vi "Sweep Control.vi"(0 "Scan control":T12=[{"Priority"=enum."Priority 1", "Scan name"=enum."OFF"}, {"Priority"=enum."Priority 0", "Scan name"=enum."DSA_freq"}, {"Priority"=enum."Priority 3", "Scan name"=enum."OFF"}, {"Priority"=enum."Priority 2", "Scan name"=enum."OFF"}], 1 "Scan parameters":T10=[{"DAQ Channel"=0, "Label"="\nappliedDC=", "Start"=-0.00372, "End"=0.00428, "Step"=5e-05, "Rate"=0.0, "VISA resource name"=""}, {"DAQ Channel"=3, "Label"="\nappliedField=", "Start"=0.3, "End"=0.0, "Step"=0.02, "Rate"=0.05, "VISA resource name"=""}, {"DAQ Channel"=3, "Label"="\nappliedVbg=", "Start"=-1.55, "End"=3.0, "Step"=0.015, "Rate"=2.0, "VISA resource name"=""}, {"DAQ Channel"=3, "Label"="\nappliedField=", "Start"=0.0, "End"=10000.0, "Step"=5000.0, "Rate"=0.0, "VISA resource name"=""}] {"Rate" format="%.2f"; "Step" format="%#_6p"; "End" format="%#_6p"; "Start" format="%#_6p"}, 3 "Comments":string="B sweep from 0.3T to 0T, 0.02T step\nDC sweep from -4mV to 4mV, 5uV step\nVbg = -5V\nVsg=40mV\nT<60mK\n\nI+/-: rightwire 1/2 200uV + DC sweep, f=9\nI2-: grounded on 4\nBase f=3\nV+/-: 5/7\nV2+/-: 4/28\nVsg: 6", 4 "Experiment folder name":string="21-SmallBsweep-DCsweep-rightdrive12-leftgrounded") -> ()   [LabVIEW 2016, in "Transport.lvclass"]
uses:
  Transport.lvclass
  Typedefs/ScanControl.ctl
  Typedefs/Cluster - ScanControl.ctl
  Typedefs/Enum - Priority.ctl
  Typedefs/Enum - Action.ctl
  Typedefs/ScanParamters.ctl
  Typedefs/Cluster - ScanParamters.ctl
  Typedefs/PostAction.ctl
  Typedefs/Enum - PostAction.ctl
  <userlib>/LevyLab/Lockin-Multichannel/Typedefs/AO-cluster.ctl
  <userlib>/LevyLab/Lockin-Multichannel/Typedefs/AO_Amp-array.ctl
  <userlib>/LevyLab/Lockin-Multichannel/Typedefs/AO_DC-array.ctl
  <userlib>/LevyLab/Lockin-Multichannel/Typedefs/AO_f-array.ctl
  <userlib>/LevyLab/Lockin-Multichannel/Typedefs/AO_phi-array.ctl
  <userlib>/LevyLab/Lockin-Multichannel/Typedefs/Function-array.ctl
  <userlib>/LevyLab/Lockin-Multichannel/Typedefs/Function-enum.ctl
  <userlib>/_OpenG.lib/array/array.llb/Empty 1D Array (Variant)__ogtk.vi
panel:
  in  "Channels: AO":T1={"AO amp (V)"=[0.0002, 0.0, 0.0, 0.0, 0.0, 0.0, 0.0, 0.0], "AO DC (V)"=[-0.004, 0.0, 0.04, 0.0, 0.0, 0.0, 0.0, 0.0], "AO f (Hz)"=[9.0, 3.0, 3.0, 3.0, 3.0, 3.0, 3.0, 3.0], "AO phi (deg)"=[0.0, 0.0, 0.0, 0.0, 0.0, 0.0, 0.0, 0.0], "function"=[enum."Sine Wave", enum."Sine Wave", enum."Sine Wave", enum."Sine Wave", enum."Sine Wave", enum."Sine Wave", enum."Sine Wave", enum."Sine Wave"]} {"AO f (Hz)" min=0.001 max=10000.0; "AO DC (V)" format="%#_6p"; "AO amp (V)" format="%#_6p"}
  in  "Experiment":enum16{"IV", "lockin_time", "Lockin_Vsg"}(ring)=enum."Lockin_Vsg"
  in  "Post action (indexing priority)":T8=[enum."Do Nothing", enum."Wait", enum."Do Nothing", enum."Do Nothing"]
  in  "Number of IV curves":i32=1
  # "if you use the lockin\nprogram remember to\nset BG/SG parameters in\n'lockin_Vsg_multichannel.vi'"
  # "Instructions: \n1, you can put multiple scan names in one priority.\n2 OFF has to put in last priority"
  # "0"
  # "1"
  # "2"
  # "3"
  # "4"
  # "5"
  # "6"
  # "7"
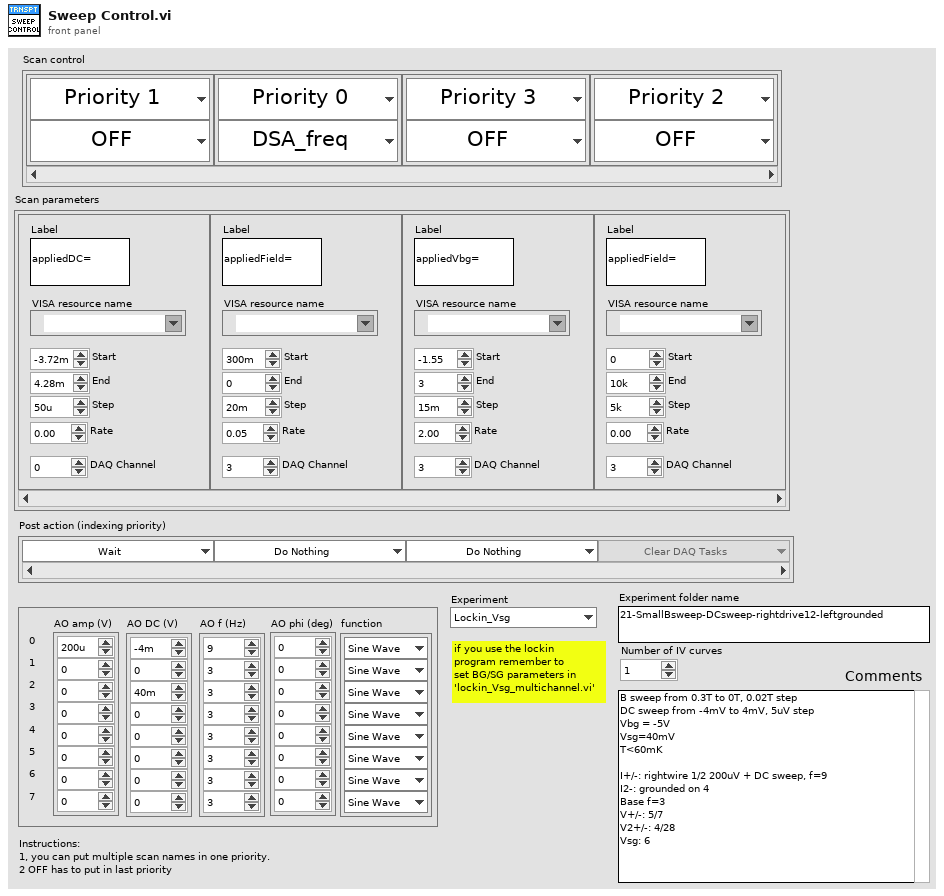
[diagram p1: front panel]
types:
  T1 = typedef "AO-cluster.ctl" = cluster{"AO amp (V)":T2, "AO DC (V)":T3, "AO f (Hz)":T4, "AO phi (deg)":T5, "function":T6}
  T2 = typedef "AO_Amp-array.ctl" = dbl[]
  T3 = typedef "AO_DC-array.ctl" = dbl[]
  T4 = typedef "AO_f-array.ctl" = dbl[]
  T5 = typedef "AO_phi-array.ctl" = dbl[]
  T6 = typedef "Function-array.ctl" = T7[]
  T7 = typedef "Function-enum.ctl" = enum16{"Sine Wave", "Triangle Wave", "Square Wave", "Sawtooth Wave"}
  T8 = typedef "Transport.lvclass/PostAction.ctl" = T9[]
  T9 = typedef "Transport.lvclass/Enum - PostAction.ctl" = enum16{"Clear DAQ Tasks", "Check Temperature", "Wait", "Do Nothing"}
  T10 = typedef "Transport.lvclass/ScanParamters.ctl" = T11[]
  T11 = typedef "Transport.lvclass/Cluster - ScanParamters.ctl" = cluster{"DAQ Channel":i32, "Label":string, "Start":dbl, "End":dbl, "Step":dbl, "Rate":dbl, "VISA resource name":refnum<visa-resource-name>}
  T12 = typedef "Transport.lvclass/ScanControl.ctl" = T13[]
  T13 = typedef "Transport.lvclass/Cluster - ScanControl.ctl" = cluster{"Priority":T14, "Scan name":T15}
  T14 = typedef "Transport.lvclass/Enum - Priority.ctl" = enum16{"Priority 0", "Priority 1", "Priority 2", "Priority 3", "Priority 4", "Priority 5"}
  T15 = typedef "Transport.lvclass/Enum - Action.ctl" = enum16{"OFF", "DSA_Vamp", "DSA_freq", "DSA_Vsg1", "DSA_Vsg2", "DSA_Vsg3", "DAQ_Vbg", "B_Field", "Humidity", "Temp", "MW_freq1", "MW_freq2", "MW_amplitude1", "MW_amplitude2"}
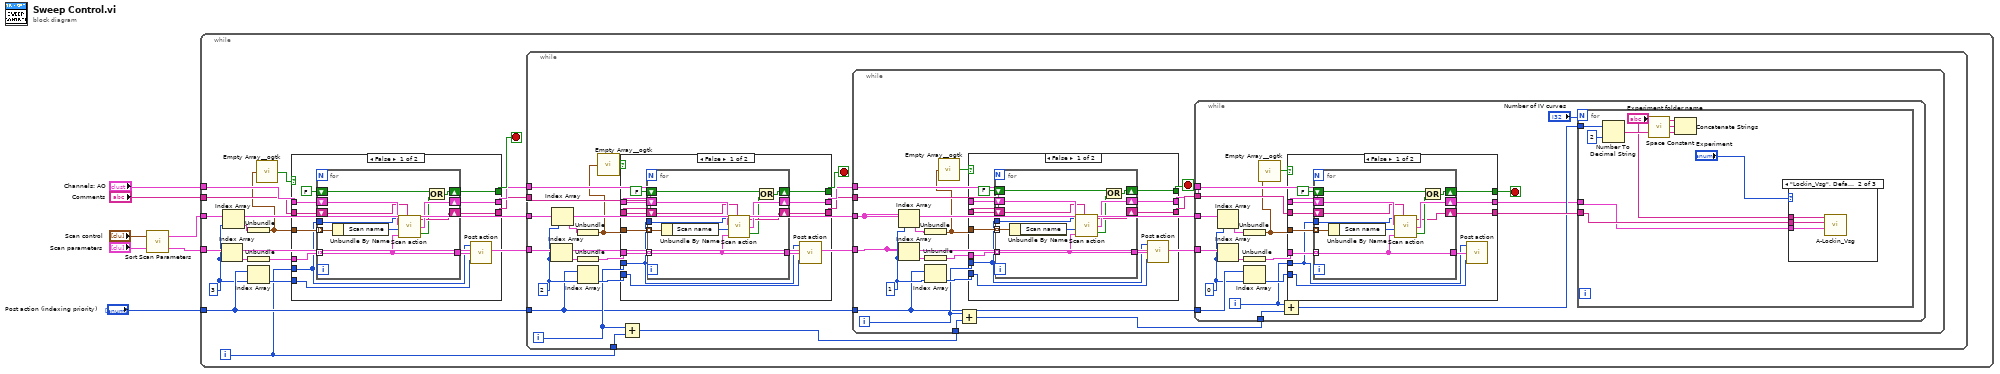
[diagram p0: block diagram]
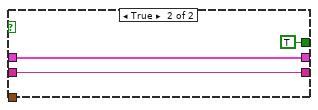
[diagram p2: hidden frame]
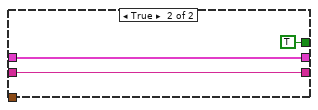
[diagram p3: hidden frame]
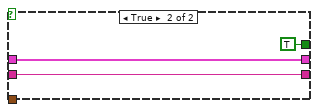
[diagram p4: hidden frame]
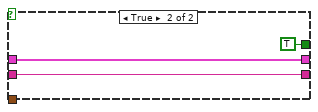
[diagram p5: hidden frame]
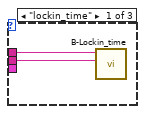
[diagram p6: hidden frame]
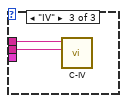
[diagram p7: hidden frame]
diagram:
  n1 = call "Sort Scan Parameters.vi"("Scan parameters"="Scan parameters", "Scan control"="Scan control") -> ("Sorted scan parameters"=w3:cluster{T10}[], "Sorted scan control"=w4:cluster{T12}[])
  n2 = while {
    tunnel: "Comments" -> [w14]
    tunnel: "Channels: AO" -> [w15]
    tunnel: w3 -> [w21]
    tunnel: w4 -> [w20]
    tunnel: "Post action (indexing priority)" -> [w16]
    i -> [w10]
    stop <- w18 stop-if-true
    w11 = 3
    n3 = Index Array(array=w21, index=w11) -> (element=w22:cluster{T10})
    n4 = Index Array(array=w20, index=w11) -> (element=w19:cluster{T12})
    n5 = Unbundle(w19) -> (w8:T12)
    n6 = Unbundle(w22) -> (w23:T10)
    n7 = Index Array(array=w16, index=w11) -> (element=w17:T9)
    n8 = call-poly <userlib>:"Empty Array__ogtk.vi"("Array"=w8) -> ("Empty Array?"=w9:bool)  [unwired: 8 in]
    n9 = case shown="False" w9 {
      tunnel: w23 -> [w34 _]
      tunnel: [w33 w47] -> w13
      tunnel: [w32 w46] -> w12
      tunnel: [w27 TRUE ("Stop?")] -> w18
      tunnel: w8 -> [w31 _]
      tunnel: w10 -> [w29 _]
      tunnel: w17 -> [w24 _]
      tunnel: w15 -> [w26 w47]
      tunnel: w14 -> [w25 w46]
      frame False {
        n10 = for {
          tunnel: w31 -> [w45] mode=indexing
          tunnel: w34 -> [w38] mode=indexing
          tunnel: w29 -> [w39]
          shift-right: [w43] -> w33
          shift-left: w26 -> [w42]
          shift-right: [w41] -> w32
          shift-left: w25 -> [w40]
          tunnel: [w38] -> w30
          shift-right: [w35] -> w27
          shift-left: FALSE -> [w37]
          n11 = Unbundle By Name(w45) -> ("Scan name"=w44:T15)
          n12 = call "Scan action.vi"("Index"=w39, "Channels: AO"=w42, "Scan control"=w44, "Scan Parameters"=w38, "Comments"=w40) -> ("Comments out"=w41:string, "Channels: AO"=w43:T1, "Stop?"=w36:bool)
          n13 = Or(x=w37, y=w36) -> (x .or. y?=w35:bool)
        }
        n14 = call "Post action.vi"("PostAction"=w24, "Scan Parameters"=w30, "Index"=w29) -> ()  [unwired: 1 in]
      }
      frame True {
      }
    }
    n15 = while {
      tunnel: w21 -> [w62]
      tunnel: w20 -> [w61]
      tunnel: w16 -> [w49]
      tunnel: w12 -> [w60]
      tunnel: w13 -> [w59]
      tunnel: w10 -> [w53]
      i -> [w54]
      stop <- w58 stop-if-true
      w55 = 2
      n16 = Index Array(array=w62, index=w55) -> (element=w65:cluster{T10})
      n17 = Index Array(array=w61, index=w55) -> (element=w66:cluster{T12})
      n18 = Unbundle(w66) -> (w50:T12)
      n19 = Unbundle(w65) -> (w64:T10)
      n20 = Index Array(array=w49, index=w55) -> (element=w63:T9)
      n21 = call-poly <userlib>:"Empty Array__ogtk.vi"("Array"=w50) -> ("Empty Array?"=w51:bool)  [unwired: 8 in]
      n22 = case shown="False" w51 {
        tunnel: w64 -> [w77 _]
        tunnel: w59 -> [w76 w91]
        tunnel: w60 -> [w75 w90]
        tunnel: [w74 w91] -> w57
        tunnel: [w73 w90] -> w56
        tunnel: [w67 TRUE ("Stop?")] -> w58
        tunnel: w50 -> [w72 _]
        tunnel: w54 -> [w69 _]
        tunnel: w63 -> [w70 _]
        frame False {
          n23 = for {
            tunnel: w72 -> [w88] mode=indexing
            tunnel: w77 -> [w81] mode=indexing
            tunnel: w69 -> [w82]
            shift-right: [w86] -> w74
            shift-left: w76 -> [w85]
            shift-right: [w84] -> w73
            shift-left: w75 -> [w83]
            tunnel: [w81] -> w71
            shift-right: [w78] -> w67
            shift-left: FALSE -> [w80]
            n24 = Unbundle By Name(w88) -> ("Scan name"=w87:T15)
            n25 = call "Scan action.vi"("Index"=w82, "Channels: AO"=w85, "Scan control"=w87, "Scan Parameters"=w81, "Comments"=w83) -> ("Comments out"=w84:string, "Channels: AO"=w86:T1, "Stop?"=w79:bool)
            n26 = Or(x=w80, y=w79) -> (x .or. y?=w78:bool)
          }
          n27 = call "Post action.vi"("PostAction"=w70, "Scan Parameters"=w71, "Index"=w69) -> ()  [unwired: 1 in]
        }
        frame True {
        }
      }
      n28 = Add(x=w54, y=w53) -> (x+y=w52:i32)
      n29 = while {
        tunnel: w57 -> [w96]
        tunnel: w56 -> [w105]
        tunnel: w61 -> [w104]
        tunnel: w62 -> [w95]
        tunnel: w49 -> [w92]
        tunnel: w52 -> [w98]
        i -> [w99]
        stop <- w101 stop-if-true
        w100 = 1
        n30 = Index Array(array=w104, index=w100) -> (element=w106:cluster{T12})
        n31 = Index Array(array=w95, index=w100) -> (element=w107:cluster{T10})
        n32 = Unbundle(w106) -> (w93:T12)
        n33 = Unbundle(w107) -> (w108:T10)
        n34 = Index Array(array=w92, index=w100) -> (element=w109:T9)
        n35 = call-poly <userlib>:"Empty Array__ogtk.vi"("Array"=w93) -> ("Empty Array?"=w94:bool)  [unwired: 8 in]
        n36 = Add(x=w99, y=w98) -> (x+y=w97:i32)
        n37 = case shown="False" w94 {
          tunnel: w108 -> [w120 _]
          tunnel: w96 -> [w119 w134]
          tunnel: w105 -> [w118 w133]
          tunnel: [w117 w134] -> w102
          tunnel: [w116 w133] -> w103
          tunnel: [w110 TRUE ("Stop?")] -> w101
          tunnel: w93 -> [w115 _]
          tunnel: w99 -> [w112 _]
          tunnel: w109 -> [w113 _]
          frame False {
            n38 = for {
              tunnel: w115 -> [w131] mode=indexing
              tunnel: w120 -> [w124] mode=indexing
              tunnel: w112 -> [w125]
              shift-right: [w129] -> w117
              shift-left: w119 -> [w128]
              shift-right: [w127] -> w116
              shift-left: w118 -> [w126]
              tunnel: [w124] -> w114
              shift-right: [w121] -> w110
              shift-left: FALSE -> [w123]
              n39 = Unbundle By Name(w131) -> ("Scan name"=w130:T15)
              n40 = call "Scan action.vi"("Index"=w125, "Channels: AO"=w128, "Scan control"=w130, "Scan Parameters"=w124, "Comments"=w126) -> ("Comments out"=w127:string, "Channels: AO"=w129:T1, "Stop?"=w122:bool)
              n41 = Or(x=w123, y=w122) -> (x .or. y?=w121:bool)
            }
            n42 = call "Post action.vi"("PostAction"=w113, "Scan Parameters"=w114, "Index"=w112) -> ()  [unwired: 1 in]
          }
          frame True {
          }
        }
        n43 = while {
          tunnel: w104 -> [w152]
          tunnel: w95 -> [w151]
          tunnel: w102 -> [w147]
          tunnel: w103 -> [w146]
          tunnel: w92 -> [w143]
          tunnel: w97 -> [w139]
          i -> [w140]
          stop <- w144 stop-if-true
          w142 = 0
          n44 = Index Array(array=w152, index=w142) -> (element=w150:cluster{T12})
          n45 = Index Array(array=w151, index=w142) -> (element=w149:cluster{T10})
          n46 = Unbundle(w150) -> (w135:T12)
          n47 = Unbundle(w149) -> (w148:T10)
          n48 = Index Array(array=w143, index=w142) -> (element=w141:T9)
          n49 = call-poly <userlib>:"Empty Array__ogtk.vi"("Array"=w135) -> ("Empty Array?"=w136:bool)  [unwired: 8 in]
          n50 = Add(x=w140, y=w139) -> (x+y=w138:i32)
          n51 = case shown="False" w136 {
            tunnel: w148 -> [w164 _]
            tunnel: w147 -> [w163 w178]
            tunnel: w146 -> [w162 w177]
            tunnel: [w161 w178] -> w137
            tunnel: [w160 w177] -> w145
            tunnel: [w155 TRUE ("Stop?")] -> w144
            tunnel: w135 -> [w159 _]
            tunnel: w140 -> [w154 _]
            tunnel: w141 -> [w157 _]
            frame False {
              n52 = for {
                tunnel: w159 -> [w175] mode=indexing
                tunnel: w164 -> [w169] mode=indexing
                tunnel: w154 -> [w170]
                shift-right: [w173] -> w161
                shift-left: w163 -> [w172]
                shift-right: [w165] -> w160
                shift-left: w162 -> [w171]
                tunnel: [w169] -> w158
                shift-right: [w166] -> w155
                shift-left: FALSE -> [w168]
                n53 = Unbundle By Name(w175) -> ("Scan name"=w174:T15)
                n54 = call "Scan action.vi"("Index"=w170, "Channels: AO"=w172, "Scan control"=w174, "Scan Parameters"=w169, "Comments"=w171) -> ("Comments out"=w165:string, "Channels: AO"=w173:T1, "Stop?"=w167:bool)
                n55 = Or(x=w168, y=w167) -> (x .or. y?=w166:bool)
              }
              n56 = call "Post action.vi"("PostAction"=w157, "Scan Parameters"=w158, "Index"=w154) -> ()  [unwired: 1 in]
            }
            frame True {
            }
          }
          n57 = for {
            N: "Number of IV curves" -> [_]
            tunnel: w137 -> [w179]
            tunnel: w145 -> [w181]
            tunnel: w138 -> [w185]
            n58 = Number To Decimal String(number=w185, width (-)=i16 2) -> (decimal integer string=w184:string)
            n59 = call <vilib>:"Space Constant.vi"() -> ("String"=w183:string)
            n60 = Concatenate Strings("Experiment folder name", w183, w184) -> ()  [unwired: 1 out]
            n61 = case shown="\"Lockin_Vsg\", Default" "Experiment" {
              tunnel: "Experiment folder name" -> [w188 w191 w193]
              tunnel: w181 -> [w187 w190 w192]
              tunnel: w179 -> [_ w189 _]
              frame "lockin_time" {
                n62 = call "B-Lockin_time.vi"("Comments"=w187, "folder name"=w188) -> ()  [unwired: 7 in, 3 out]
              }
              frame "Lockin_Vsg", Default {
                n63 = call "A-Lockin_Vsg.vi"("Channels: AO"=w189, "Comments"=w190, "ITX folder"=w191) -> ()  [unwired: 9 in]
              }
              frame "IV" {
                n64 = call "C-IV.vi"("Notes 2"=w192, "Experiment folder name"=w193) -> ()  [unwired: 8 in, 2 out]
              }
            }
          }
        }
      }
    }
  }
